vi "UMLEditor IsMouseOutsideDrawingArea.vi"(0 "Mouse":T1, 1 "Draw Area Size":cluster{"Width":u32, "Height":u32}, 2 "Origin":cluster{"Horizontal":i16, "Vertical":i16}) -> (14 "OutsideDrawingArea":bool)   [LabVIEW 2016]
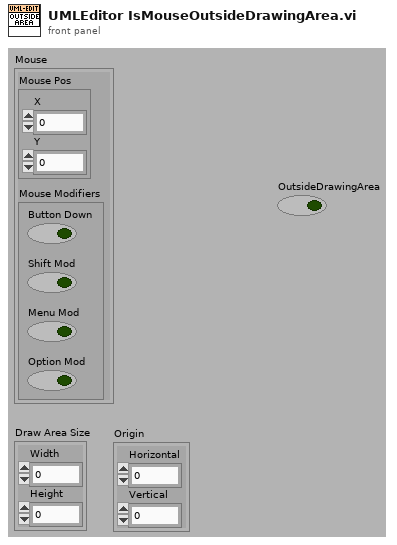
[diagram p1: front panel]
types:
  T1 = cluster{"Mouse Pos":cluster{"X":i32, "Y":i32}, "Mouse Modifiers":cluster{"Button Down":bool, "Shift Mod":bool, "Menu Mod":bool, "Option Mod":bool}}
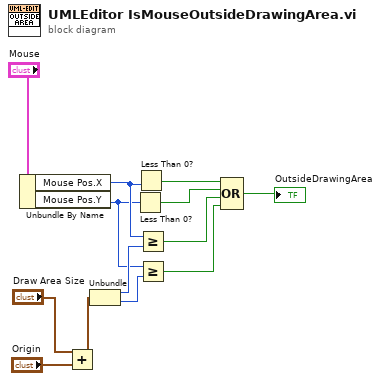
[diagram p0: block diagram]
diagram:
  n1 = Unbundle By Name("Mouse") -> ("Mouse Pos.X"=w13:i32, "Mouse Pos.Y"=w8:i32)
  n2 = Add(x="Draw Area Size", y="Origin") -> (x+y=w1:cluster{u32, u32})
  n3 = Unbundle(w1) -> (w9:u32, w7:u32)
  n4 = Less Than 0?(x=w8) -> (x < 0?=w10:bool)
  n5 = Less Than 0?(x=w13) -> (x < 0?=w11:bool)
  n6 = Greater Or Equal?(x=w13, y=w9) -> (x >= y?=w6:bool)
  n7 = Greater Or Equal?(x=w8, y=w7) -> (x >= y?=w5:bool)
  n8 = Compound Arithmetic op=OR(w11, w10, w6, w5) -> (→"OutsideDrawingArea":bool)
